vi "Build Configuration Data.vi"(8 "error in (no error)":errorcluster, 11 "Configuration Window in":refnum<class "Configuration Window.lvclass">) -> (0 "error out":errorcluster, 2 "Configuration":T1={"Language"={"Name"=""}, "Path Config"={"Data Folder Path"=path "", "PNG Folder Path"=path "", "mp3 Folder Path"=path ""}, "Image Viewer Config"={"Center Point"={"Size"=3, "Color"=0, "Show?"=FALSE}, "bp Point"={"Size"=3, "Color"=0, "Show?"=FALSE}, "w Point"={"Size"=3, "Color"=0, "Show?"=FALSE}, "b Box"={"Fill Color"=0, "Border Color"=0, "Show?"=FALSE}, "i Box"={"Fill Color"=0, "Border Color"=0, "Show?"=FALSE}, "o Point"={"Size"=3, "Color"=0, "Show?"=FALSE}, "c Point"={"Size"=3, "Color"=0, "Show?"=FALSE}}}, 3 "Configuration Window out":refnum<class "Configuration Window.lvclass">)   [LabVIEW 2018, in "Configuration Window.lvlib" / "Configuration Window.lvclass"]
uses:
  Configuration Window.lvclass
  Main Panel/LF2R IDE/Const Configuration.ctl
  Main Panel/LF2R IDE/Const Path Setting.ctl
  Main Panel/LF2R IDE/Const Image Viewer Setting.ctl
  Configuration Window.lvclass/Configuration Window.ctl
  Main Panel/LF2R IDE/Main Panel.lvclass
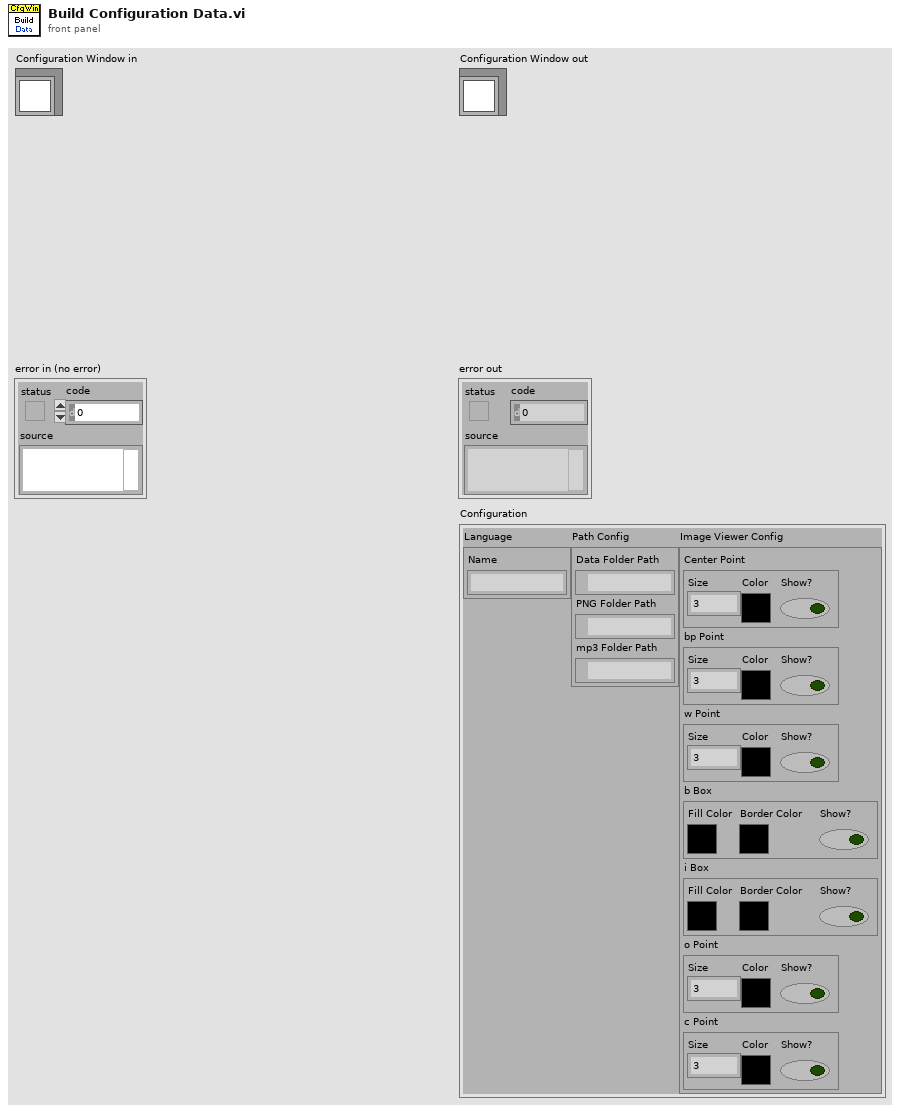
[diagram p1: front panel]
types:
  T1 = typedef "Main Panel.lvlib/Main Panel.lvclass/Const Configuration.ctl" = cluster{"Language":cluster{"Name":string}, "Path Config":T2, "Image Viewer Config":T3}
  T2 = typedef "Main Panel.lvlib/Main Panel.lvclass/Const Path Setting.ctl" = cluster{"Data Folder Path":path, "PNG Folder Path":path, "mp3 Folder Path":path}
  T3 = typedef "Main Panel.lvlib/Main Panel.lvclass/Const Image Viewer Setting.ctl" = cluster{"Center Point":cluster{"Size":i32, "Color":u32, "Show?":bool}, "bp Point":cluster{"Size":i32, "Color":u32, "Show?":bool}, "w Point":cluster{"Size":i32, "Color":u32, "Show?":bool}, "b Box":cluster{"Fill Color":u32, "Border Color":u32, "Show?":bool}, "i Box":cluster{"Fill Color":u32, "Border Color":u32, "Show?":bool}, "o Point":cluster{"Size":i32, "Color":u32, "Show?":bool}, "c Point":cluster{"Size":i32, "Color":u32, "Show?":bool}}
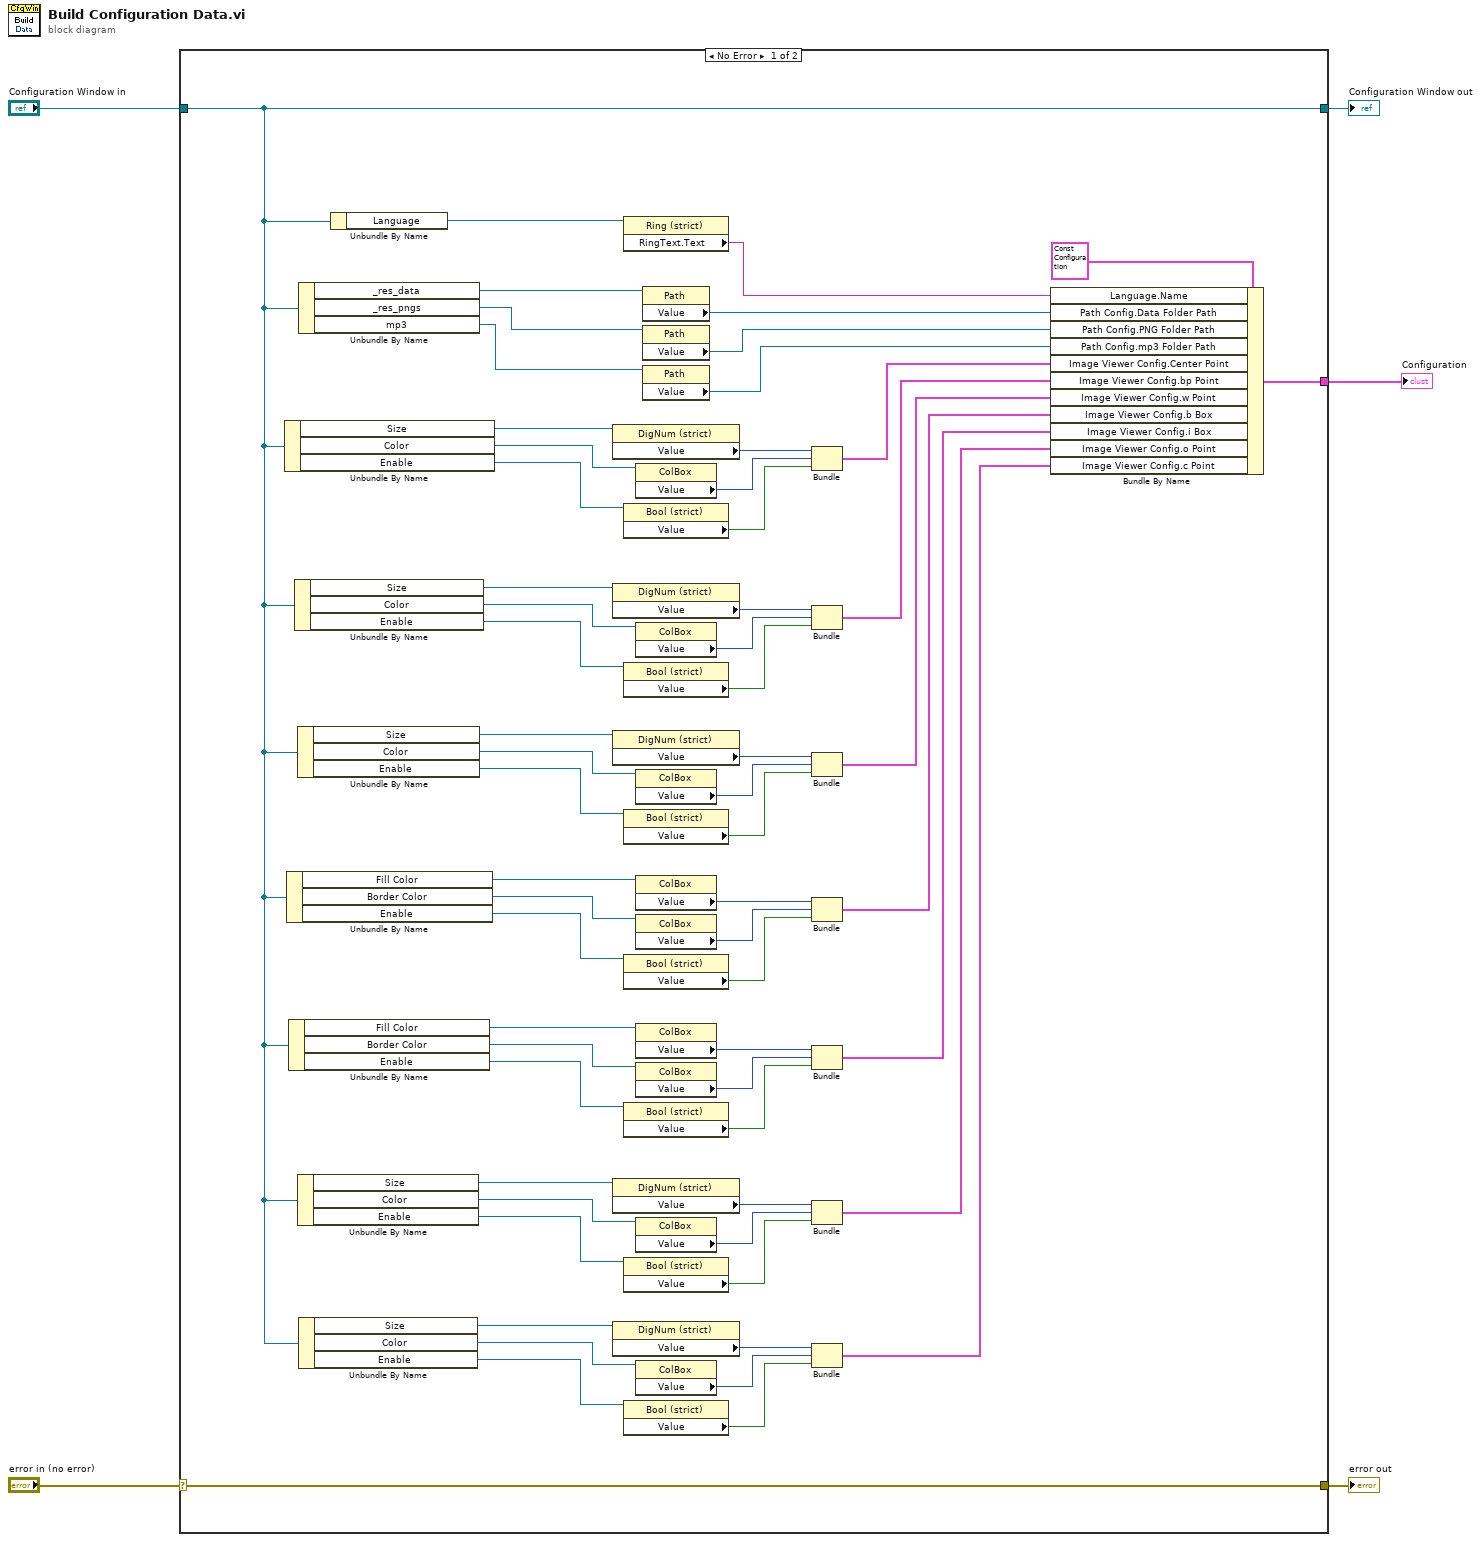
[diagram p0: block diagram]
diagram:
  n1 = case shown="No Error" "error in (no error)" {
    selector: "error in (no error)" -> [w66 w68]
    tunnel: [w66 w68] -> w4
    tunnel: [w10 w67] -> w2
    tunnel: "Configuration Window in" -> [w10 w67]
    tunnel: [w11 _] -> w1
    frame No Error {
      n2 = Unbundle By Name(w10) -> ("Size"=w60:refnum<vi>, "Color"=w59:refnum<vi>, "Enable"=w58:refnum<vi>)
      n3 = Unbundle By Name(w10) -> ("Fill Color"=w36:refnum<vi>, "Border Color"=w35:refnum<vi>, "Enable"=w34:refnum<vi>)
      n4 = Unbundle By Name(w10) -> ("Fill Color"=w32:refnum<vi>, "Border Color"=w28:refnum<vi>, "Enable"=w27:refnum<vi>)
      n5 = Unbundle By Name(w10) -> ("Size"=w48:refnum<vi>, "Color"=w49:refnum<vi>, "Enable"=w50:refnum<vi>)
      n6 = Unbundle By Name(w10) -> ("Size"=w46:refnum<vi>, "Color"=w42:refnum<vi>, "Enable"=w41:refnum<vi>)
      n7 = Unbundle By Name(w10) -> ("Size"=w22:refnum<vi>, "Color"=w21:refnum<vi>, "Enable"=w20:refnum<vi>)
      n8 = Unbundle By Name(w10) -> ("_res_data"=w65:refnum<vi>, "_res_pngs"=w62:refnum<vi>, "mp3"=w7:refnum<vi>)
      n9 = Unbundle By Name(w10) -> ("Size"=w18:refnum<vi>, "Color"=w14:refnum<vi>, "Enable"=w13:refnum<vi>)
      n10 = Unbundle By Name(w10) -> ("Language"=w9:refnum<vi>)
      n11 = property class="DigNum (strict)"(reference=w60) -> ("Value"=w57:i32)  [unwired: 1 in, 2 out]
      n12 = property class="DigNum (strict)"(reference=w48) -> ("Value"=w51:i32)  [unwired: 1 in, 2 out]
      n13 = property class="DigNum (strict)"(reference=w46) -> ("Value"=w45:i32)  [unwired: 1 in, 2 out]
      n14 = property class="DigNum (strict)"(reference=w22) -> ("Value"=w23:i32)  [unwired: 1 in, 2 out]
      n15 = property class="DigNum (strict)"(reference=w18) -> ("Value"=w17:i32)  [unwired: 1 in, 2 out]
      n16 = property class="Ring (strict)"(reference=w9) -> ("RingText.Text"=w8:string)  [unwired: 1 in, 2 out]
      n17 = property class="Bool (strict)"(reference=w58) -> ("Value"=w55:bool)  [unwired: 1 in, 2 out]
      n18 = property class="Bool (strict)"(reference=w50) -> ("Value"=w53:bool)  [unwired: 1 in, 2 out]
      n19 = property class="Bool (strict)"(reference=w41) -> ("Value"=w43:bool)  [unwired: 1 in, 2 out]
      n20 = property class="Bool (strict)"(reference=w34) -> ("Value"=w39:bool)  [unwired: 1 in, 2 out]
      n21 = property class="Bool (strict)"(reference=w27) -> ("Value"=w29:bool)  [unwired: 1 in, 2 out]
      n22 = property class="Bool (strict)"(reference=w20) -> ("Value"=w25:bool)  [unwired: 1 in, 2 out]
      n23 = property class="Bool (strict)"(reference=w13) -> ("Value"=w15:bool)  [unwired: 1 in, 2 out]
      n24 = property class="ColBox"(reference=w59) -> ("Value"=w56:u32)  [unwired: 1 in, 2 out]
      n25 = property class="ColBox"(reference=w49) -> ("Value"=w52:u32)  [unwired: 1 in, 2 out]
      n26 = property class="ColBox"(reference=w42) -> ("Value"=w44:u32)  [unwired: 1 in, 2 out]
      n27 = property class="ColBox"(reference=w36) -> ("Value"=w37:u32)  [unwired: 1 in, 2 out]
      n28 = property class="ColBox"(reference=w35) -> ("Value"=w38:u32)  [unwired: 1 in, 2 out]
      n29 = property class="ColBox"(reference=w32) -> ("Value"=w31:u32)  [unwired: 1 in, 2 out]
      n30 = property class="ColBox"(reference=w28) -> ("Value"=w30:u32)  [unwired: 1 in, 2 out]
      n31 = property class="ColBox"(reference=w21) -> ("Value"=w24:u32)  [unwired: 1 in, 2 out]
      n32 = property class="ColBox"(reference=w14) -> ("Value"=w16:u32)  [unwired: 1 in, 2 out]
      n33 = property class="Path"(reference=w65) -> ("Value"=w63:path)  [unwired: 1 in, 2 out]
      n34 = property class="Path"(reference=w62) -> ("Value"=w61:path)  [unwired: 1 in, 2 out]
      n35 = property class="Path"(reference=w7) -> ("Value"=w6:path)  [unwired: 1 in, 2 out]
      n36 = Bundle("Value"=w57, "Value"=w56, "Value"=w55) -> (w54:cluster{"Value":i32, "Value":u32, "Value":bool})  [unwired: 1 in]
      n37 = Bundle("Value"=w51, "Value"=w52, "Value"=w53) -> (w47:cluster{"Value":i32, "Value":u32, "Value":bool})  [unwired: 1 in]
      n38 = Bundle("Value"=w45, "Value"=w44, "Value"=w43) -> (w40:cluster{"Value":i32, "Value":u32, "Value":bool})  [unwired: 1 in]
      n39 = Bundle("Value"=w37, "Value"=w38, "Value"=w39) -> (w33:cluster{"Value":u32, "Value":u32, "Value":bool})  [unwired: 1 in]
      n40 = Bundle("Value"=w31, "Value"=w30, "Value"=w29) -> (w26:cluster{"Value":u32, "Value":u32, "Value":bool})  [unwired: 1 in]
      n41 = Bundle("Value"=w23, "Value"=w24, "Value"=w25) -> (w19:cluster{"Value":i32, "Value":u32, "Value":bool})  [unwired: 1 in]
      n42 = Bundle("Value"=w17, "Value"=w16, "Value"=w15) -> (w12:cluster{"Value":i32, "Value":u32, "Value":bool})  [unwired: 1 in]
      n43 = Bundle By Name(cluster=T1 {"Language"={"Name"=""}, "Path Config"={"Data Folder Path"=path "", "PNG Folder Path"=path "", "mp3 Folder Path"=path ""}, "Image Viewer Config"={"Center Point"={"Size"=3, "Color"=0, "Show?"=FALSE}, "bp Point"={"Size"=3, "Color"=0, "Show?"=FALSE}, "w Point"={"Size"=3, "Color"=0, "Show?"=FALSE}, "b Box"={"Fill Color"=0, "Border Color"=0, "Show?"=FALSE}, "i Box"={"Fill Color"=0, "Border Color"=0, "Show?"=FALSE}, "o Point"={"Size"=3, "Color"=0, "Show?"=FALSE}, "c Point"={"Size"=3, "Color"=0, "Show?"=FALSE}}} ("Configuration 2"), "Language.Name"=w8, "Path Config.Data Folder Path"=w63, "Path Config.PNG Folder Path"=w61, "Path Config.mp3 Folder Path"=w6, "Image Viewer Config.Center Point"=w54, "Image Viewer Config.bp Point"=w47, "Image Viewer Config.w Point"=w40, "Image Viewer Config.b Box"=w33, "Image Viewer Config.i Box"=w26, "Image Viewer Config.o Point"=w19, "Image Viewer Config.c Point"=w12) -> (w11:T1)
    }
    frame Error {
    }
  }
  "error out" <- w4
  "Configuration Window out" <- w2
  "Configuration" <- w1
